vi "Load ProtoFile.vi"(0 "protoFile ref in":u64, 1 "File Base path":path, 2 "File Name":string, 3 "error in (no error)":errorcluster) -> (7 "protoFile ref out":u64, 10 "error out":errorcluster)   [LabVIEW 2019, in "gRPC Template Creation Utility.lvlib"]
uses:
  gRPC Template Creation Utility.lvlib
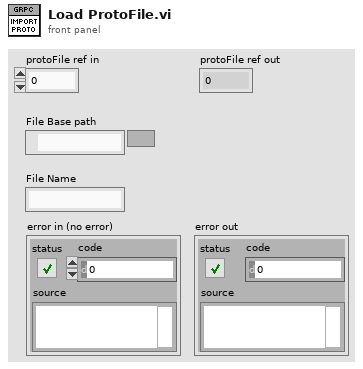
[diagram p1: front panel]
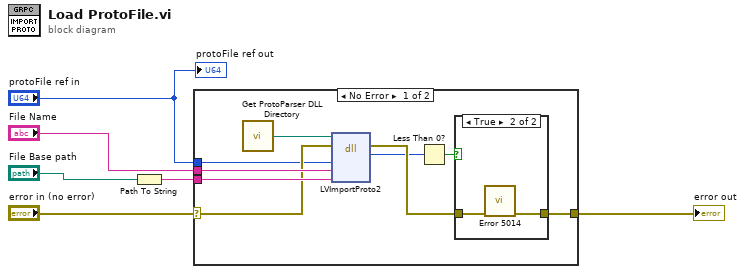
[diagram p0: block diagram]
diagram:
  n1 = Path To String(path="File Base path") -> (string=w6:string)
  n2 = case shown="No Error" "error in (no error)" {
    selector: "error in (no error)" -> [w13 w19]
    tunnel: w6 -> [w15 _]
    tunnel: "File Name" -> [w14 _]
    tunnel: [w10 w19] -> w2
    tunnel: "protoFile ref in" -> [w7 _]
    frame No Error {
      n3 = call "Get ProtoParser DLL Directory.vi"() -> ("Proto Parser Directory"=w12:path)
      n4 = dll-call lib="?" fn="LVImportProto2"(path in=w12, error in=w13, "protoRef"=w7, "protoName"=w14, "SearchPaths"=w15) -> (error out=w11:errorcluster, "return type"=w9:i32)  [unwired: 4 in, 1 out]
      n5 = Less Than 0?(x=w9) -> (x < 0?=w8:bool)
      n6 = case shown="True" w8 {
        tunnel: w11 -> [w16 w18]
        tunnel: [w16 w17] -> w10
        frame False {
        }
        frame True {
          n7 = call "Error 5014.vi"("error in (no error)"=w18) -> ("error out"=w17:errorcluster)  [unwired: 10 in]
        }
      }
    }
    frame Error {
    }
  }
  "error out" <- w2
  "protoFile ref out" <- "protoFile ref in"
